vi "Execute.vi"(8 "error in (no error)":errorcluster, 11 "Node in":refnum<class "bt_Composite.lvclass">) -> (0 "error out":errorcluster, 1 "Status":T1, 3 "Node out":refnum<class "bt_Composite.lvclass">)   [LabVIEW 2021, in "BT.lvlib" / "bt_Composite.lvclass"]
uses:
  bt_Composite.lvclass
  abs_Node/Status.ctl
  bt_Composite.lvclass/bt_Composite.ctl
  Properties/Read Index.vi
  abs_Node/bt_Node.lvclass
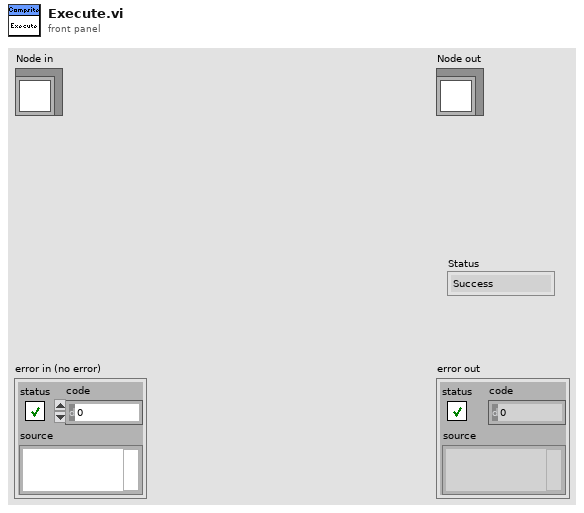
[diagram p1: front panel]
types:
  T1 = typedef "BT.lvlib/bt_Node.lvclass/Status.ctl" = enum16{"Success", "Failure", "Running"}
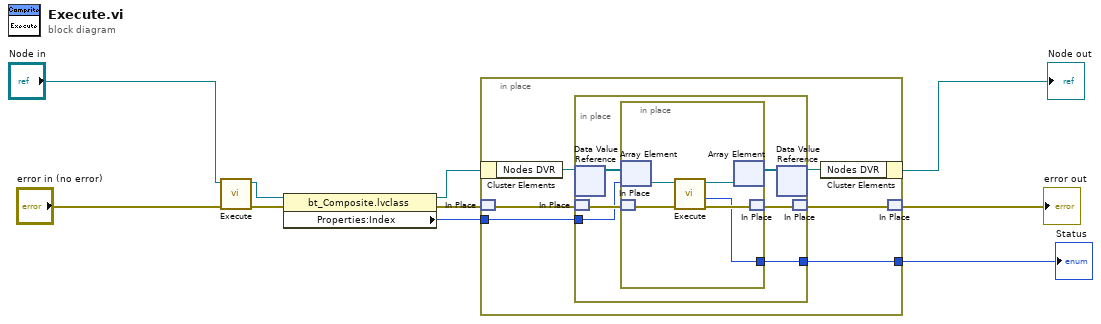
[diagram p0: block diagram]
diagram:
  n1 = call-parent "Execute.vi"("error in (no error)"="error in (no error)", "Node in"="Node in") -> ("error out"=w5:errorcluster, "Node out"=w3:refnum<class "bt_Composite.lvclass">)  [unwired: 7 in, 1 out]
  n2 = property class="bt_Composite.lvclass"(reference=w3, error in=w5) -> (reference out=w2:refnum<class "bt_Composite.lvclass">, error out=w4:errorcluster, "Properties:Index"=w1:i32)
  n3 = in-place {
    in-place-border: [w12] -> w6
    in-place-border: w1 -> [w11]
    n4 = in-place-cluster #1(w2) -> ("Nodes DVR"=w16:refnum<data-value>)
    n5 = in-place-match #2(w4) -> (w14:errorcluster)
    n6 = in-place {
      in-place-border: [w18] -> w12
      in-place-border: w11 -> [w17]
      n7 = in-place-dvr #3(w16) -> (w22:refnum<class "bt_Node.lvclass">[])  [unwired: 1 out]
      n8 = in-place-match #4(w14) -> (w20:errorcluster)
      n9 = in-place {
        in-place-border: [w23] -> w18
        n10 = in-place-array #5(w22, w17) -> (w27:refnum<class "bt_Node.lvclass">)
        n11 = in-place-match #6(w20) -> (w25:errorcluster)
        n12 = call-dynamic "Execute.vi"("error in (no error)"=w25, "Node in"=w27) -> ("error out"=w24:errorcluster, "Status"=w23:T1, "Node out"=w26:refnum<class "bt_Node.lvclass">)  [unwired: 7 in]
        n13 = in-place-array #5(w26) -> (w21:refnum<class "bt_Node.lvclass">[])  [unwired: 1 out]
        n14 = in-place-match #6(w24) -> (w19:errorcluster)
      }
      n15 = in-place-dvr #3(w21) -> (w15:refnum<data-value>)  [unwired: 1 out]
      n16 = in-place-match #4(w19) -> (w13:errorcluster)
    }
    n17 = in-place-cluster #1("Nodes DVR"=w15) -> (→"Node out":refnum<class "bt_Composite.lvclass">)
    n18 = in-place-match #2(w13) -> (→"error out":errorcluster)
  }
  "Status" <- w6
